vi "探头型号.vi"(11 "校准参数":u16(ring) caption="校准参数：" items=["pH", "DO", "浊度", "电导率", "叶绿素a", "藻密度", "ORP", "COD", "DO2", "氯化物", "氨氮", "水中油", "悬浮物"]) -> (3 "探头型号":T1=enum."纳清", 5 "禁用项[]":i32[](array[numeric]), 7 "value":i32)   [LabVIEW 2016, in "斯坦道多参数.lvlib"]
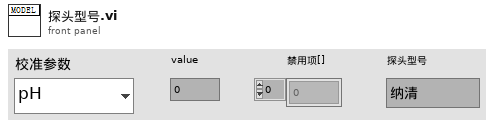
[diagram p1: front panel]
types:
  T1 = typedef "斯坦道多参数.lvlib/探头类型.ctl" = enum16{"禹山", "国弘", "纳清", "STD"}
  T2 = cluster{"pH探头选择":T1, "DO探头选择":T1, "电导率探头选择":T1, "浊度探头选择":T1, "悬浮物探头选择":T1, "叶绿素a探头选择":T1, "蓝绿藻探头选择":T1, "orp探头选择":T1, "COD探头选择":T1, "DO2探头选择":T1, "氨氮探头选择":T1, "水中油探头选择":T1, "余氯探头选择":T1}
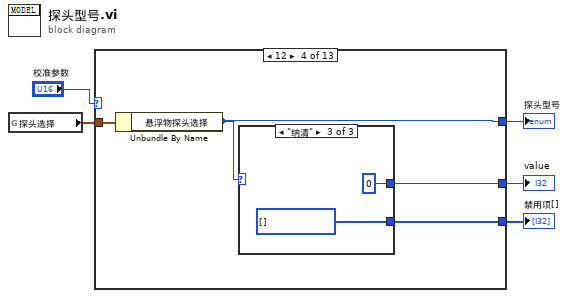
[diagram p0: block diagram]
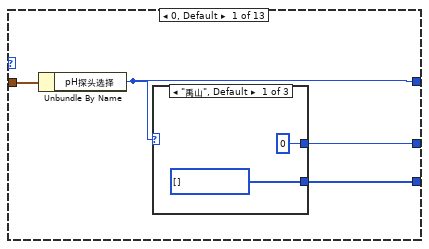
[diagram p2: hidden frame]
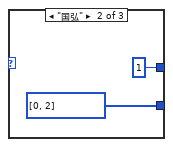
[diagram p3: hidden frame]
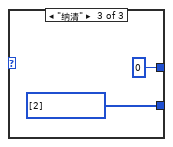
[diagram p4: hidden frame]
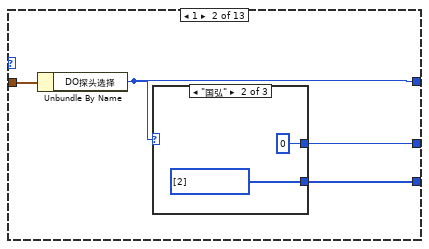
[diagram p5: hidden frame]
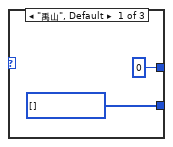
[diagram p6: hidden frame]
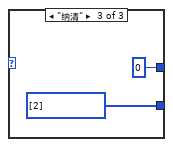
[diagram p7: hidden frame]
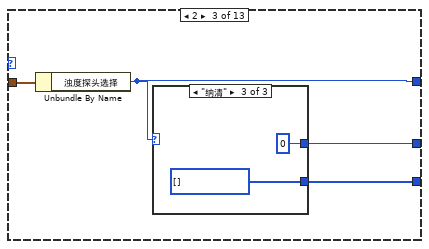
[diagram p8: hidden frame]
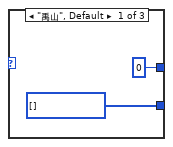
[diagram p9: hidden frame]
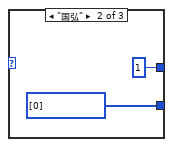
[diagram p10: hidden frame]
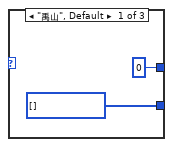
[diagram p11: hidden frame]
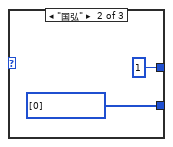
[diagram p12: hidden frame]
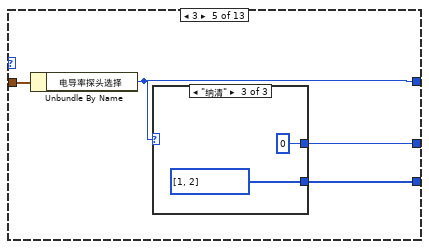
[diagram p13: hidden frame]
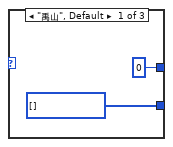
[diagram p14: hidden frame]
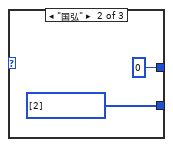
[diagram p15: hidden frame]
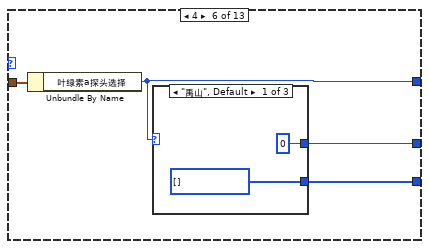
[diagram p16: hidden frame]
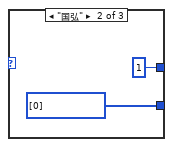
[diagram p17: hidden frame]
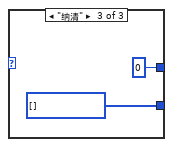
[diagram p18: hidden frame]
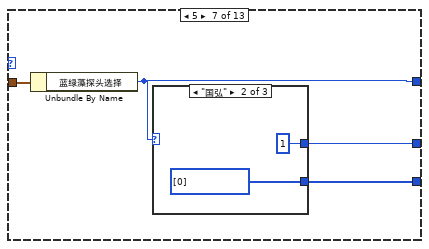
[diagram p19: hidden frame]
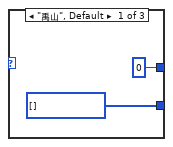
[diagram p20: hidden frame]
diagram:
  n1 = global read "断电保存变量.vi" "探头选择"() -> (w4:T2)
  n2 = case shown="12" "校准参数" {
    tunnel: w4 -> [w9 w19 w29 w39 w49 w59 w69 w79 w83 w93 _ w100 _]
    tunnel: [w8 w18 w28 w38 w48 w58 w68 w78 w82 w92 u16 1 ("DO2探头选择") w99 u16 1 ("DO2探头选择")] -> w3
    tunnel: [w7 w17 w27 w37 w47 w57 w67 i32[] [0, 10, 20] ("禁用项[]") w81 i32[] [] ("禁用项[]") i32[] [2] ("禁用项[]") i32[] [2] ("禁用项[]") i32[] [] ("禁用项[]")] -> w2
    tunnel: [w6 w16 w26 w36 w46 w56 w66 0 w80 0 0 0 0] -> w1
    frame 0, Default {
      n3 = Unbundle By Name(w9) -> ("pH探头选择"=w8:T1)
      n4 = case shown="\"禹山\", Default" w8 {
        tunnel: [i32[] [] ("禁用项[]") i32[] [0, 2] ("禁用项[]") i32[] [2] ("禁用项[]")] -> w7
        tunnel: [0 1 0] -> w6
        frame "禹山", Default {
        }
        frame "国弘" {
        }
        frame "纳清" {
        }
      }
    }
    frame 1 {
      n5 = Unbundle By Name(w19) -> ("DO探头选择"=w18:T1)
      n6 = case shown="\"国弘\"" w18 {
        tunnel: [i32[] [] ("禁用项[]") i32[] [2] ("禁用项[]") i32[] [2] ("禁用项[]")] -> w17
        tunnel: [0 0 0] -> w16
        frame "禹山", Default {
        }
        frame "国弘" {
        }
        frame "纳清" {
        }
      }
    }
    frame 2 {
      n7 = Unbundle By Name(w29) -> ("浊度探头选择"=w28:T1)
      n8 = case shown="\"纳清\"" w28 {
        tunnel: [i32[] [] ("禁用项[]") i32[] [0] ("禁用项[]") i32[] [] ("禁用项[]")] -> w27
        tunnel: [0 1 0] -> w26
        frame "禹山", Default {
        }
        frame "国弘" {
        }
        frame "纳清" {
        }
      }
    }
    frame 12 {
      n9 = Unbundle By Name(w39) -> ("悬浮物探头选择"=w38:T1)
      n10 = case shown="\"纳清\"" w38 {
        tunnel: [i32[] [] ("禁用项[]") i32[] [0] ("禁用项[]") i32[] [] ("禁用项[]")] -> w37
        tunnel: [0 1 0] -> w36
        frame "禹山", Default {
        }
        frame "国弘" {
        }
        frame "纳清" {
        }
      }
    }
    frame 3 {
      n11 = Unbundle By Name(w49) -> ("电导率探头选择"=w48:T1)
      n12 = case shown="\"纳清\"" w48 {
        tunnel: [i32[] [] ("禁用项[]") i32[] [2] ("禁用项[]") i32[] [1, 2] ("禁用项[]")] -> w47
        tunnel: [0 0 0] -> w46
        frame "禹山", Default {
        }
        frame "国弘" {
        }
        frame "纳清" {
        }
      }
    }
    frame 4 {
      n13 = Unbundle By Name(w59) -> ("叶绿素a探头选择"=w58:T1)
      n14 = case shown="\"禹山\", Default" w58 {
        tunnel: [i32[] [] ("禁用项[]") i32[] [0] ("禁用项[]") i32[] [] ("禁用项[]")] -> w57
        tunnel: [0 1 0] -> w56
        frame "禹山", Default {
        }
        frame "国弘" {
        }
        frame "纳清" {
        }
      }
    }
    frame 5 {
      n15 = Unbundle By Name(w69) -> ("蓝绿藻探头选择"=w68:T1)
      n16 = case shown="\"国弘\"" w68 {
        tunnel: [i32[] [] ("禁用项[]") i32[] [0] ("禁用项[]") i32[] [] ("禁用项[]")] -> w67
        tunnel: [0 1 0] -> w66
        frame "禹山", Default {
        }
        frame "国弘" {
        }
        frame "纳清" {
        }
      }
    }
    frame 6 {
      n17 = Unbundle By Name(w79) -> ("orp探头选择"=w78:T1)
    }
    frame 7 {
      n18 = Unbundle By Name(w83) -> ("COD探头选择"=w82:T1)
      n19 = case shown="\"禹山\", Default" w82 {
        tunnel: [i32[] [] ("禁用项[]") i32[] [0] ("禁用项[]") i32[] [] ("禁用项[]")] -> w81
        tunnel: [0 1 0] -> w80
        frame "禹山", Default {
        }
        frame "国弘" {
        }
        frame "纳清" {
        }
      }
    }
    frame 8 {
      n20 = Unbundle By Name(w93) -> ("DO2探头选择"=w92:T1)
    }
    frame 9 {
    }
    frame 10 {
      n21 = Unbundle By Name(w100) -> ("氨氮探头选择"=w99:T1)
    }
    frame 11 {
    }
  }
  "探头型号" <- w3
  "禁用项[]" <- w2
  "value" <- w1
